vi "moveSingleStep.vi"(1 "direction":i32, 2 "motorSpeed":dbl, 3 "VISA resource name":refnum<visa-resource-name>) -> (0 "position":dbl format="%#.3g")   [LabVIEW 2013]
panel:
  out "currentPos":dbl caption="Current Position (mm)" format="%.3g"
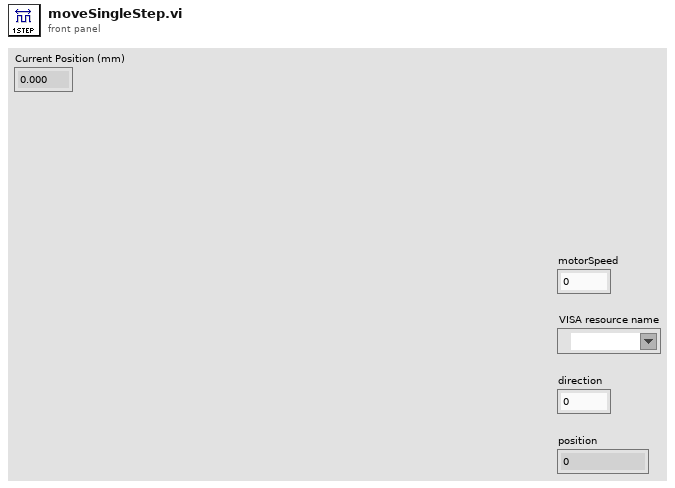
[diagram p1: front panel]
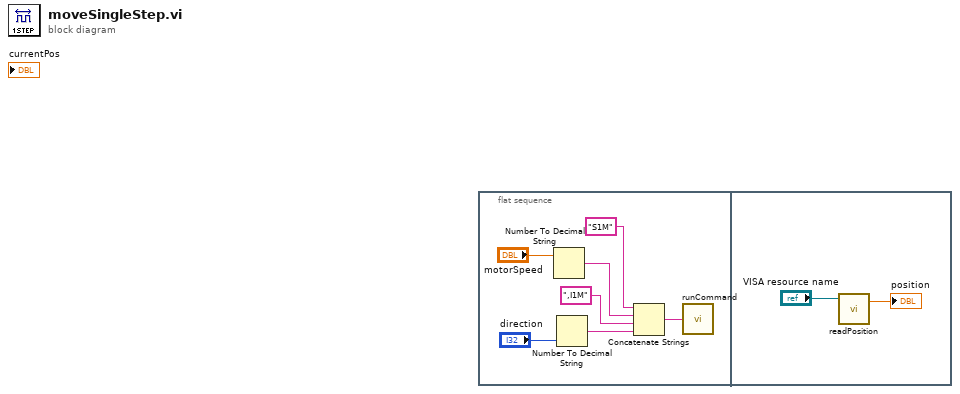
[diagram p0: block diagram]
diagram:
  n1 = flat-sequence {
    frame #0 {
      n2 = Number To Decimal String(number="motorSpeed") -> (decimal integer string=w2:string)  [unwired: 1 in]
      n3 = Number To Decimal String(number="direction") -> (decimal integer string=w4:string)  [unwired: 1 in]
      n4 = Concatenate Strings("S1M" ("command"), w2, ",I1M" ("command"), w4) -> (w6:string)
      n5 = call "runCommand.vi"("command"=w6) -> ()  [unwired: 1 in]
    }
    frame #1 {
      n6 = call "readPosition.vi"("VISA resource name"="VISA resource name") -> ("position"=→"position":dbl)  [unwired: 1 in, 2 out]
    }
  }
